vi "Select_RTM.vi"() -> ()   [LabVIEW 2020]
panel:
  in  "stop":bool
  in  "Menu":bool
  # "Menu #1"
  # "Menu #2"
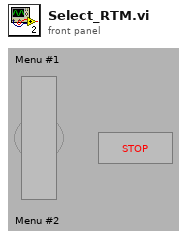
[diagram p1: front panel]
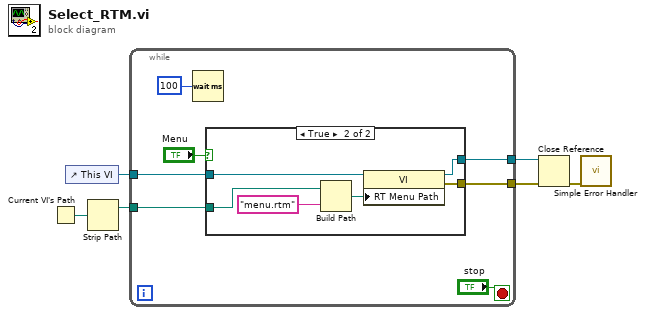
[diagram p0: block diagram]
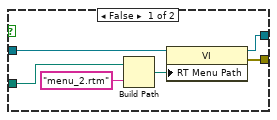
[diagram p2: hidden frame]
diagram:
  n1 = Current VI's Path() -> (path=w3:path)
  n2 = control-ref of="This VI"() -> (w6:refnum<vi>)
  n3 = Strip Path(path=w3) -> (stripped path=w2:path)  [unwired: 1 out]
  n4 = while {
    tunnel: w6 -> [w12]
    tunnel: [w11] -> w5
    tunnel: [w10] -> w4
    tunnel: w2 -> [w7]
    stop <- "stop" stop-if-true
    n5 = Wait (ms)(milliseconds to wait=u32 100) -> ()  [unwired: 1 out]
    n6 = case shown="True" "Menu" {
      tunnel: w12 -> [w19 w25]
      tunnel: [w18 w24] -> w11
      tunnel: [w17 w23] -> w10
      tunnel: w7 -> [w15 w20]
      frame False {
        n7 = Build Path(base path=w15, name or relative path="menu_2.rtm") -> (appended path=w14:path)
        n8 = property class="VI"(reference=w19, "RT Menu Path"=w14) -> (reference out=w18:refnum<vi>, error out=w17:errorcluster)  [unwired: 1 in]
      }
      frame True {
        n9 = Build Path(base path=w20, name or relative path="menu.rtm") -> (appended path=w21:path)
        n10 = property class="VI"(reference=w25, "RT Menu Path"=w21) -> (reference out=w24:refnum<vi>, error out=w23:errorcluster)  [unwired: 1 in]
      }
    }
  }
  n11 = Close Reference(reference=w5, error in (no error)=w4) -> (error out=w1:errorcluster)
  n12 = call <vilib>:"Simple Error Handler.vi"("error in (no error)"=w1) -> ()  [unwired: 4 in, 5 out]
